vi "increment rep1.vi"(4 "State":i16, 5 "Time":dbl format="%.2f", 6 "Sensor Values":dbl[](array[numeric]), 7 "Set Points":dbl[](array[numeric])) -> (0 "required data":T1={"Set Point names"=["reset state", "state to increment", "slope", "intercept", "max x", "reps"], "required number of setpoints"=6, "required number of sensors"=0, "Sensor names"=[]}, 3 "output value":dbl)   [LabVIEW 2019]
panel:
  # "Enter the correct information for this control code in the required data structure below. Then make the current value default by right clicking on the border of the data structure. Select \"data operations\" and then select \"make current value default\". These values will be displayed by process controller."
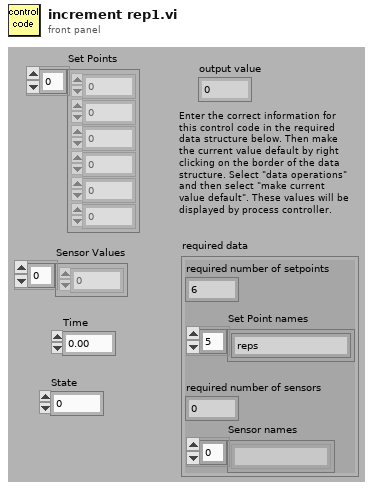
[diagram p1: front panel]
types:
  T1 = cluster{"Set Point names":string[], "required number of setpoints":u8, "required number of sensors":u8, "Sensor names":string[]}
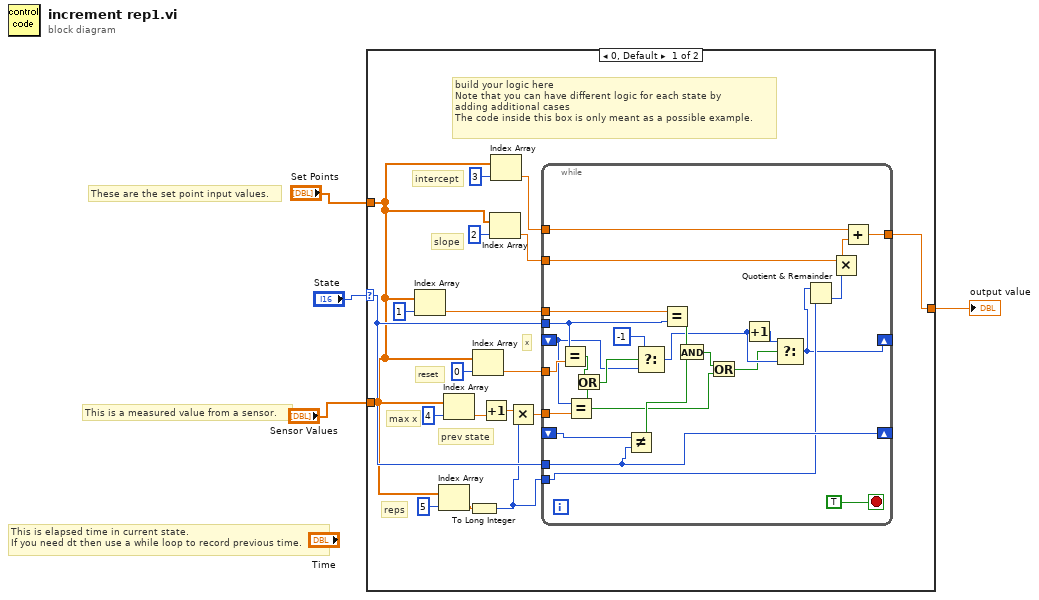
[diagram p0: block diagram]
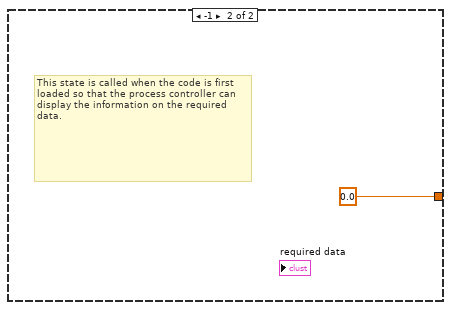
[diagram p2: hidden frame]
diagram:
  # "These are the set point input values."
  # "This is a measured value from a sensor."
  # "This is elapsed time in current state.\nIf you need dt then use a while loop to record previous time."
  n1 = case shown="0, Default" "State" {
    selector: "State" -> [w19 _]
    tunnel: [w15 0.0 ("fraction on")] -> w3
    tunnel: "Set Points" -> [w10 _]
    tunnel: "Sensor Values" -> [_ _]
    frame 0, Default {
      # "reps"
      # "max x"
      # "prev state"
      # "reset"
      # "intercept"
      # "slope"
      # "x"
      # "build your logic here\nNote that you can have different logic for each state by\nadding additional cases\nThe code inside this box is only meant as a possible example."
      n2 = Index Array(array=w10, index=1) -> (element=w20:dbl)
      n3 = Index Array(array=w10, index=5) -> (element=w9:dbl)
      n4 = Index Array(array=w10, index=4) -> (element=w7:dbl)
      n5 = To Long Integer(number=w9) -> (32bit integer=w8:i32)
      n6 = Index Array(array=w10, index=0) -> (element=w13:dbl)
      n7 = Increment(x=w7) -> (x+1=w6:dbl)
      n8 = Index Array(array=w10, index=2) -> (element=w17:dbl)
      n9 = Index Array(array=w10, index=3) -> (element=w16:dbl)
      n10 = Multiply(x=w6, y=w8) -> (x*y=w5:dbl)
      n11 = while {
        shift-right: [w46] -> _
        shift-left: _ -> [w34]
        tunnel: w19 -> [w46]
        tunnel: w20 -> [w47]
        tunnel: w19 -> [w37]
        shift-right: [w24] -> _
        shift-left: _ -> [w30]
        tunnel: w17 -> [w41]
        tunnel: w16 -> [w44]
        tunnel: [w43] -> w15
        tunnel: w13 -> [w36]
        tunnel: w5 -> [w33]
        tunnel: w8 -> [w25]
        stop <- TRUE stop-if-true
        n12 = Equal?(x=w37, y=w36) -> (x = y?=w32:bool)
        n13 = Equal?(x=w30, y=w33) -> (x = y?=w27:bool)
        n14 = Or(x=w32, y=w27) -> (x .or. y?=w31:bool)
        n15 = Not Equal?(x=w34, y=w46) -> (x != y?=w45:bool)
        n16 = Select(t=-1, s=w31, f=w30) -> (s? t:f=w35:i32)
        n17 = Equal?(x=w47, y=w37) -> (x = y?=w40:bool)
        n18 = And(x=w40, y=w45) -> (x .and. y?=w28:bool)
        n19 = Or(x=w28, y=w27) -> (x .or. y?=w26:bool)
        n20 = Increment(x=w35) -> (x+1=w39:i32)
        n21 = Select(t=w39, s=w26, f=w35) -> (s? t:f=w24:i32)
        n22 = Quotient & Remainder(x=w24, y=w25) -> (floor(x/y)=w23:i32)  [unwired: 1 out]
        n23 = Multiply(x=w41, y=w23) -> (x*y=w38:dbl)
        n24 = Add(x=w44, y=w38) -> (x+y=w43:dbl)
      }
    }
    frame -1 {
      # "This state is called when the code is first loaded so that the process controller can display the information on the required data."
    }
  }
  "output value" <- w3
